vi "Clear SystErr Queue.vi"(8 "error":errorcluster, 11 "VISA":refnum<visa-resource-name>) -> (0 "error out":errorcluster, 3 "VISA out":refnum<visa-resource-name>)   [LabVIEW 2019, in "TDK-Lambda GEN LAN Series.lvlib"]
doc: "Clears the power supply output message buffers. \n\nIf a response is waiting in the output buffer, this VI will read the message to clear the buffer. \nIf any errors are in the SYSTEM:ERROR message buffer, this VI will send \"SYST:ERR:ENAB\" to clear the error messages."
uses:
  <instrlib>/TDK-Lambda GEN LAN Series/TDK-Lambda GEN LAN Series.lvlib
panel:
  # "Clear SYST:ERR Queue"
  # "TDK-Lambda Genesys \n LAN\n  DC Power Supplies"
  # "Clears left-over messages in\nSYSTEM:ERROR queue.\nErrors and responses are discarded"
  # "(c) 2019 TDK-Lambda.  ALL RIGHTS RESERVED."
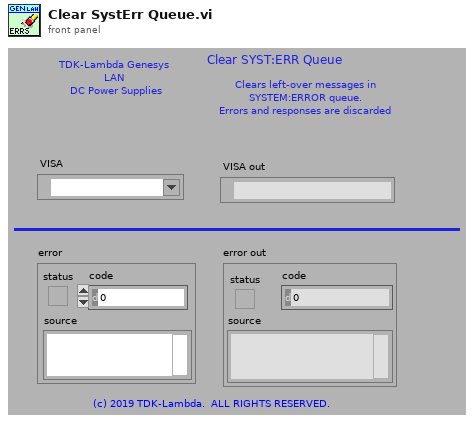
[diagram p1: front panel]
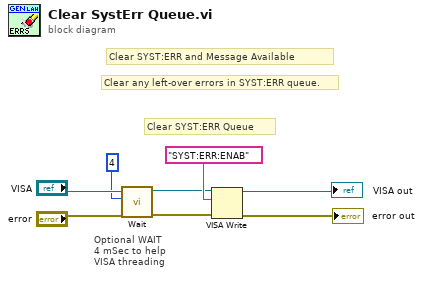
[diagram p0: block diagram]
diagram:
  # "Optional WAIT \n4 mSec to help VISA threading"
  # "Clear SYST:ERR Queue"
  # "Clear any left-over errors in SYST:ERR queue."
  # "Clear SYST:ERR and Message Available"
  n1 = call <instrlib>:"Wait.vi"("error"="error", "Delay (20 mS)"=u32 4, "VISA"="VISA") -> ("error out"=w4:errorcluster, "VISA out"=w5:refnum<visa-resource-name>)  [unwired: 7 in]
  n2 = VISA Write(VISA resource name=w5, write buffer="SYST:ERR:ENAB", error in (no error)=w4) -> (VISA resource name out=→"VISA out":refnum<visa-resource-name>, error out=→"error out":errorcluster)  [unwired: 1 out]
